vi "HXG2_Digital-IN.vi"(8 "error in (no error)":errorcluster, 10 "FreqMdot Task In":refnum<k21>, 11 "DIG IN TASK":refnum<k21>) -> (0 "error out":errorcluster, 2 "Mdot (lbm/hr)":dbl, 3 "Digital In":T1)   [LabVIEW 2012]
uses:
  Controls/HXG2_DigitalIn.ctl
  <vilib>/DAQmx/read.llb/DAQmx Read (Counter DBL 1Chan 1Samp).vi
  <vilib>/DAQmx/read.llb/DAQmx Read (Digital 1D Bool NChan 1Samp 1Line).vi
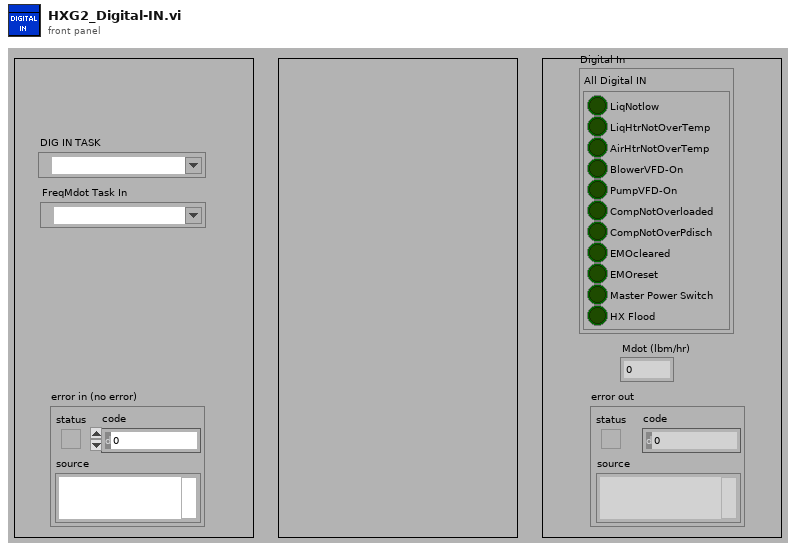
[diagram p1: front panel]
types:
  T1 = typedef "HXG2_DigitalIn.ctl" = cluster{"All Digital IN":cluster{"LiqNotlow":bool, "LiqHtrNotOverTemp":bool, "AirHtrNotOverTemp":bool, "BlowerVFD-On":bool, "PumpVFD-On":bool, "CompNotOverloaded":bool, "CompNotOverPdisch":bool, "EMOcleared":bool, "EMOreset":bool, "Master Power Switch":bool, "HX Flood":bool}}
  T2 = cluster{"data[0]":bool, "data[1]":bool, "data[2]":bool, "data[3]":bool, "data[4]":bool, "data[5]":bool, "data[6]":bool, "data[7]":bool, "data[8]":bool, "data[9]":bool, "data[10]":bool}
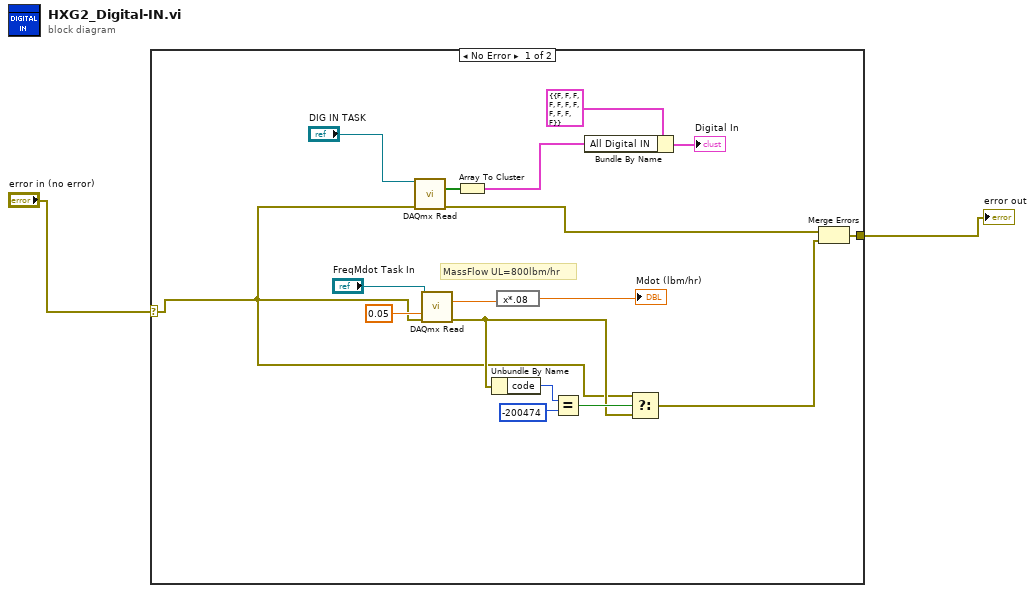
[diagram p0: block diagram]
diagram:
  n1 = case shown="No Error" "error in (no error)" {
    selector: "error in (no error)" -> [w4 w20]
    tunnel: [w3 w20] -> w1
    frame No Error {
      # "MassFlow UL=800lbm/hr"
      n2 = call-poly <vilib>:"DAQmx Read.vi"("task/channels in"="DIG IN TASK", "error in"=w4) -> ("data"=w18:bool[], "error out"=w14:errorcluster)  [unwired: 11 in, 1 out]
      n3 = call-poly <vilib>:"DAQmx Read.vi"("task/channels in"="FreqMdot Task In", "timeout"=0.05, "error in"=w4) -> ("data"=w12:dbl, "error out"=w6:errorcluster)  [unwired: 10 in, 1 out]
      n4 = Array To Cluster(array=w18) -> (cluster=w15:T2)
      n5 = Unbundle By Name(w6) -> ("code"=w8:i32)
      n6 = expression code="x*.08"(w12) -> (→"Mdot (lbm/hr)":dbl)
      n7 = Equal?(x=w8, y=-200474) -> (x = y?=w7:bool)
      n8 = Bundle By Name(cluster=T1 {"All Digital IN"={"LiqNotlow"=FALSE, "LiqHtrNotOverTemp"=FALSE, "AirHtrNotOverTemp"=FALSE, "BlowerVFD-On"=FALSE, "PumpVFD-On"=FALSE, "CompNotOverloaded"=FALSE, "CompNotOverPdisch"=FALSE, "EMOcleared"=FALSE, "EMOreset"=FALSE, "Master Power Switch"=FALSE, "HX Flood"=FALSE}} ("Digital In"), "All Digital IN"=w15) -> (→"Digital In":T1)
      n9 = Select(t=w4, s=w7, f=w6) -> (s? t:f=w5:errorcluster)
      n10 = Merge Errors(w14, w5) -> (w3:errorcluster)
    }
    frame Error {
    }
  }
  "error out" <- w1
